vi "3.4.vi"(2 "尾":string, 3 "数值":dbl, 4 "头":string) -> (0 "字符串长度":i32, 1 "连接后的字符串":string)   [LabVIEW 2017]
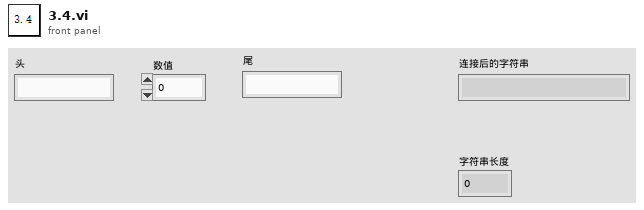
[diagram p1: front panel]
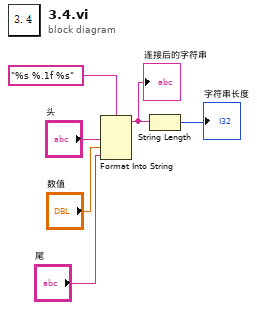
[diagram p0: block diagram]
diagram:
  n1 = Format Into String(format string="%s %.1f %s" ("格式字符串"), "头", "数值", "尾") -> (resulting string=w3:string)  [unwired: 2 in, 1 out]
  "连接后的字符串" <- w3
  n2 = String Length(string=w3) -> (length=→"字符串长度":i32)
